vi "lab1_example_usrp_sine_signal_generator.vi"() -> ()   [LabVIEW 2014]
uses:
  <vilib>/measure/maspectr.llb/Power Spectrum and PSD Export Mode.ctl
  <vilib>/Analysis/1siggen.llb/Ramp Pattern by Samples.vi
  sub_var_stop.vi
  <instrlib>/niUSRP/niUSRP Fetch Rx Data (CDB Cluster).vi
  <vilib>/measure/maspectr.llb/FFT Power Spectrum and PSD for 1 Chan (CDB).vi
  <instrlib>/niUSRP/niUSRP Write Tx Data (CDB Cluster).vi
  <vilib>/Analysis/NI_AALBase.lvlib
  <vilib>/measure/NI_MAPro.lvlib
panel:
  out "coerced gain":dbl format="%#_6f"
  in  "number of samples":i64=20000
  out "coerced carrier frequency":dbl=915000000.0 format="%#_6p"
  out "coerced IQ rate":dbl=200000.0 format="%#_6p"
  in  "gain 2":dbl format="%#_6f"
  in  "gain":dbl format="%#_6f"
  in  "carrier frequency":dbl=915000000.0 format="%#_6p"
  in  "IQ rate":dbl=200000.0 format="%#_6p"
  in  "device names 2":refnum<k15>="192.168.10.2"
  in  "device names":refnum<k15>="192.168.10.2"
  out "Power Spectrum graph":cluster{"f0":dbl, "df":dbl, "magnitude":dbl[]}(graph)={"f0"=-0.5, "df"=5e-05, "magnitude"=[]}
  out "Sine wave":dbl[](graph)
  in  "duration":dbl=0.02 format="%#_13g"
  in  "frequency":dbl=10000.0 format="%#_13g"
  in  "stop":bool
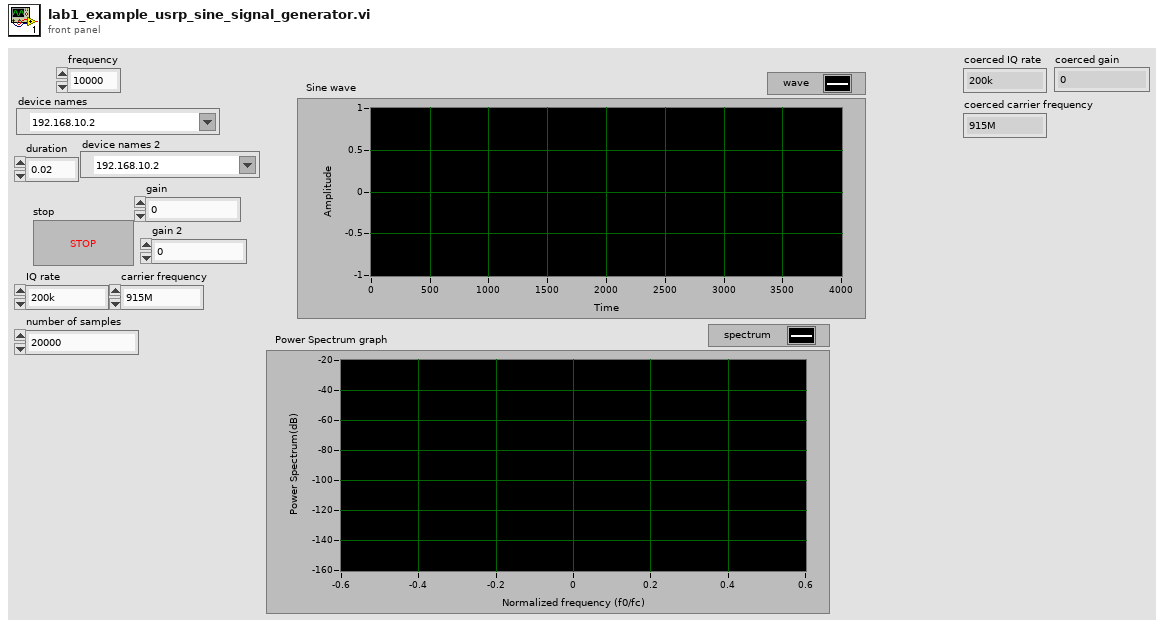
[diagram p1: front panel]
types:
  T1 = typedef "NI_MAPro.lvlib/Power Spectrum and PSD Export Mode.ctl" = u16
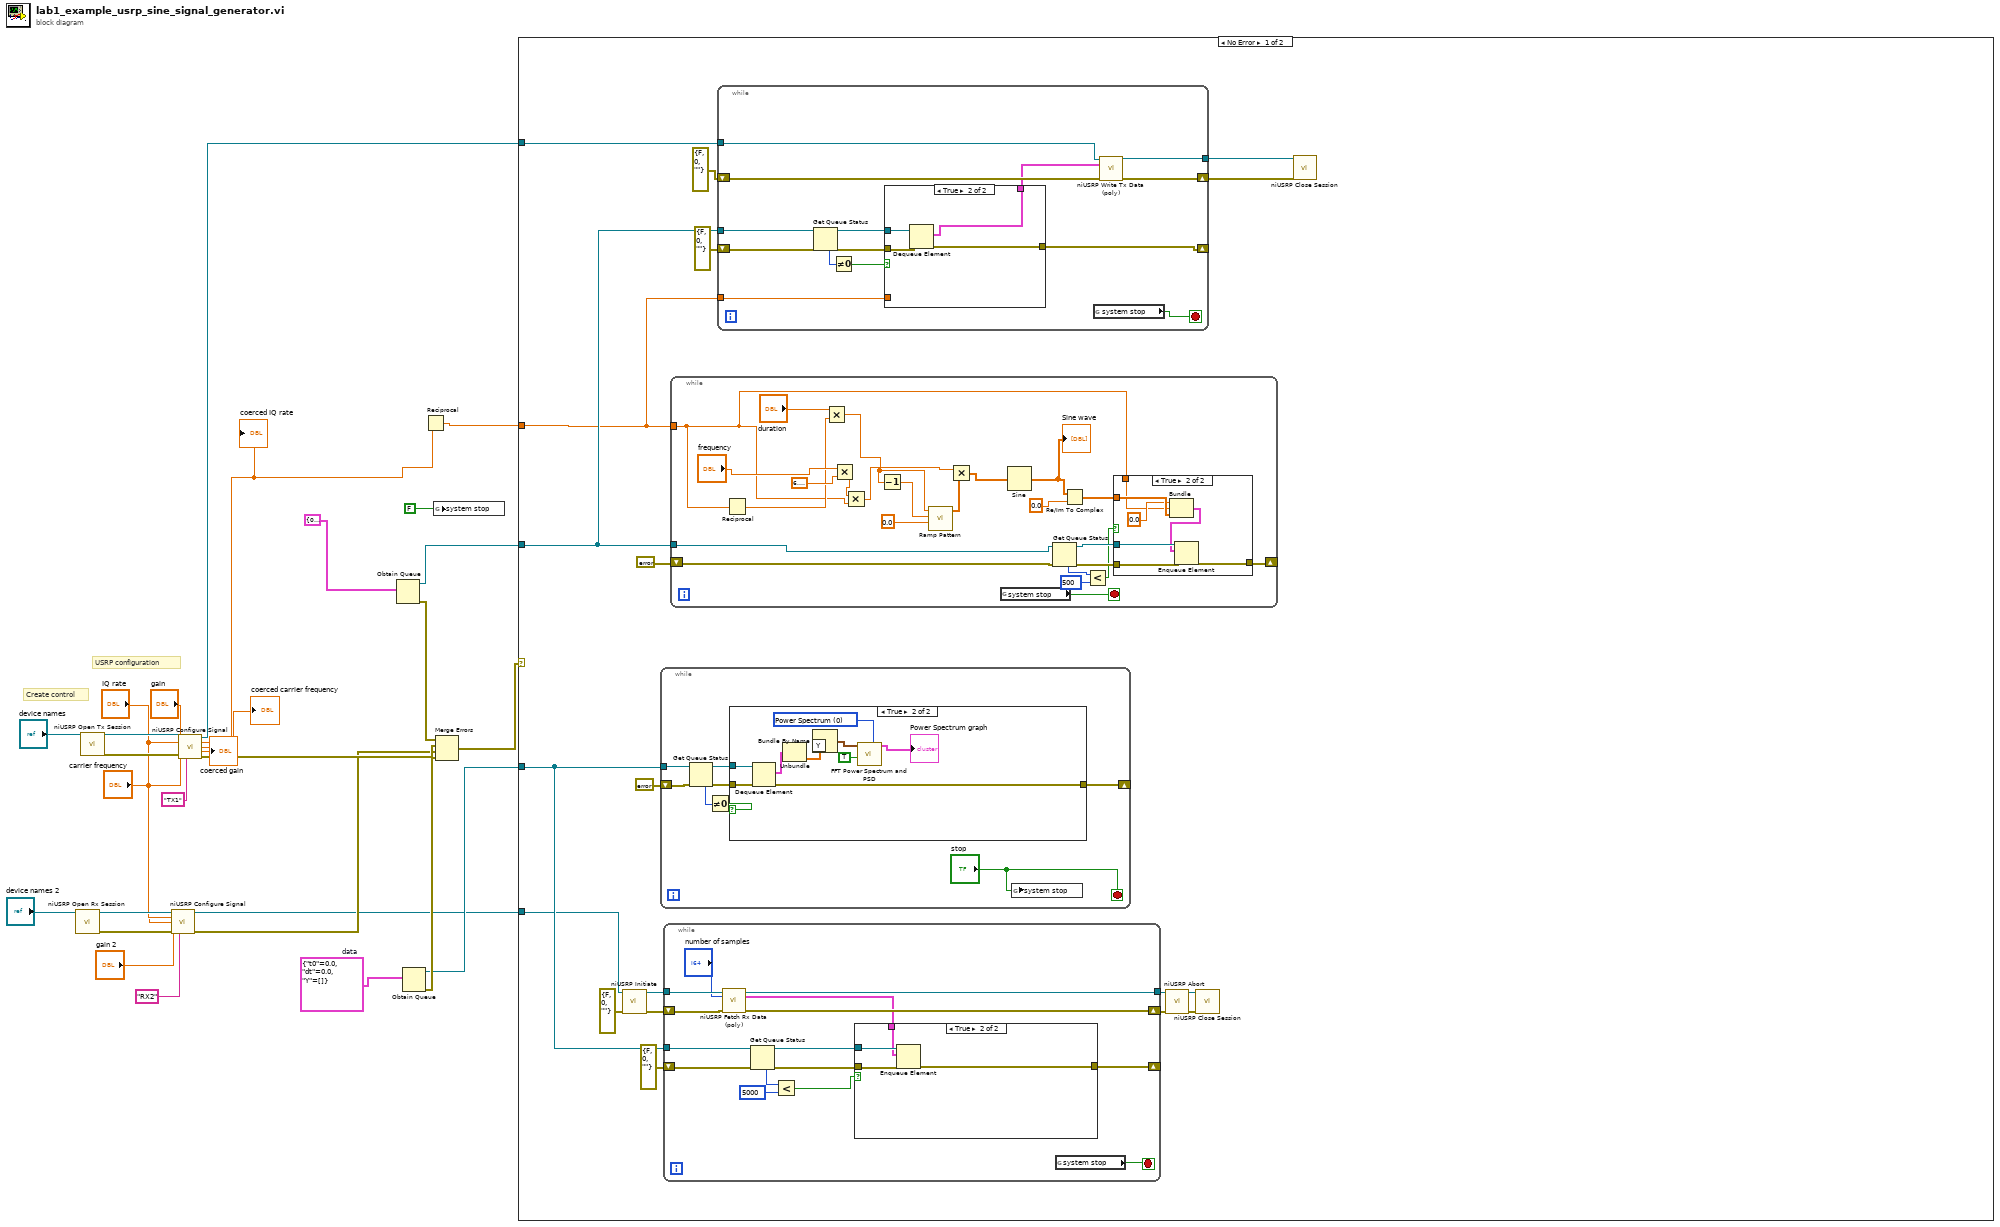
[diagram p0: block diagram]
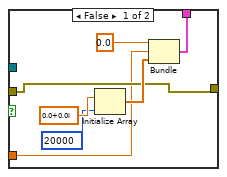
[diagram p3: hidden frame]
diagram:
  w9 = cluster{"t0":dbl, "dt":dbl, "Y":cdb[]} {"t0"=0.0, "dt"=0.0, "Y"=[]}  # data
  # "Create control"
  # "USRP configuration"
  n1 = call <instrlib>:"niUSRP Open Rx Session.vi"("device names"="device names 2") -> ("session handle out"=w24:refnum<k15>, "error out"=w23:errorcluster)  [unwired: 13 in]
  n2 = call <instrlib>:"niUSRP Open Tx Session.vi"("device names"="device names") -> ("session handle out"=w26:refnum<k15>, "error out"=w25:errorcluster)  [unwired: 13 in]
  n3 = call <instrlib>:"niUSRP Configure Signal.vi"("session handle"=w24, "IQ rate"="IQ rate", "carrier frequency"="carrier frequency", "gain"="gain 2", "error in (no error)"=w23, "active antenna"="RX2") -> ("session handle out"=w6:refnum<k15>, "error out"=w12:errorcluster)  [unwired: 5 in, 3 out]
  n4 = call <instrlib>:"niUSRP Configure Signal.vi"("session handle"=w26, "IQ rate"="IQ rate", "carrier frequency"="carrier frequency", "gain"="gain", "error in (no error)"=w25, "active antenna"="TX1") -> ("session handle out"=w5:refnum<k15>, "coerced IQ rate"=w2:dbl, "coerced carrier frequency"=→"coerced carrier frequency":dbl, "coerced gain"=→"coerced gain":dbl, "error out"=w13:errorcluster)  [unwired: 5 in]
  "coerced IQ rate" <- w2
  n5 = Obtain Queue(element data type=cluster{"t0":dbl, "dt":dbl, "Y":cdb[]} {"t0"=0.0, "dt"=1.0, "Y"=[]} ("data")) -> (queue out=w27:refnum<queue>, error out=w14:errorcluster)  [unwired: 4 in, 1 out]
  n6 = Obtain Queue(element data type=w9) -> (queue out=w7:refnum<queue>, error out=w8:errorcluster)  [unwired: 4 in, 1 out]
  n7 = Reciprocal(x=w2) -> (1/x=w4:dbl)
  n8 = global write "sub_var_stop.vi" "system stop"(FALSE) -> ()
  n9 = Merge Errors(w14, w13, w12, w8) -> (w10:errorcluster)
  n10 = case shown="No Error" w10 {
    tunnel: w27 -> [w31 _]
    tunnel: w7 -> [w35 _]
    tunnel: w6 -> [w33 _]
    tunnel: w5 -> [w32 _]
    tunnel: w4 -> [w29 _]
    frame No Error {
      n11 = call <instrlib>:"niUSRP Initiate.vi"("session handle"=w33, "error in (no error)"=errorcluster {"status"=FALSE, "code"=0, "source"=""}) -> ("session handle out"=w43:refnum<k15>, "error out"=w42:errorcluster)  [unwired: 12 in]
      n12 = while {
        tunnel: w35 -> [w99]
        shift-right: [w93] -> _
        shift-left: errorcluster {"status"=FALSE, "code"=0, "source"=""} ("error out") -> [w98]
        stop <- "stop" stop-if-true
        n13 = Get Queue Status(queue=w99, error in (no error)=w98) -> (queue out=w95:refnum<queue>, error out=w94:errorcluster, # elements in queue=w97:i32)  [unwired: 1 in, 5 out]
        n14 = Not Equal To 0?(x=w97) -> (x != 0?=w96:bool)
        n15 = case shown="True" w96 {
          tunnel: w95 -> [_ w110]
          tunnel: w94 -> [w101 w109]
          tunnel: [w101 w108] -> w93
          frame False {
          }
          frame True {
            w104 = T1 0 items=["Power Spectrum", "Power Spectral Density"] ("export mode")
            n16 = Dequeue Element(queue=w110, error in (no error)=w109) -> (element=w103:cluster{"t0":dbl, "dt":dbl, "Y":cdb[]}, error out=w108:errorcluster)  [unwired: 1 in, 2 out]
            n17 = Unbundle "Unbundle"(w103) -> ("Y"=w102:cdb[])  [unwired: 2 out]
            n18 = Bundle By Name("Y"=w102) -> (w107:waveform(cdb))  [unwired: 1 in]
            n19 = call-poly <vilib>:"FFT Power Spectrum and PSD.vi"("export mode"=w104, "dB On (F)"=TRUE, "time signal"=w107) -> ("Power Spectrum / PSD"=→"Power Spectrum graph":cluster{"f0":dbl, "df":dbl, "magnitude":dbl[]})  [unwired: 5 in, 3 out]
          }
        }
        n20 = global write "sub_var_stop.vi" "system stop"("stop") -> ()
      }
      n21 = while {
        tunnel: w43 -> [w61]
        shift-right: [w57] -> w39
        shift-left: w42 -> [w60]
        tunnel: [w58] -> w38
        tunnel: w35 -> [w56]
        shift-right: [w48] -> _
        shift-left: errorcluster {"status"=FALSE, "code"=0, "source"=""} ("error out") -> [w55]
        stop <- w62 stop-if-true
        n22 = call-poly <instrlib>:"niUSRP Fetch Rx Data (poly).vi"("session handle"=w61, "number of samples"="number of samples", "error in (no error)"=w60) -> ("session handle out"=w58:refnum<k15>, "data"=w49:cluster{"t0":dbl, "dt":dbl, "Y":cdb[]}, "error out"=w57:errorcluster)  [unwired: 9 in, 1 out]
        n23 = Get Queue Status(queue=w56, error in (no error)=w55) -> (queue out=w51:refnum<queue>, error out=w50:errorcluster, # elements in queue=w54:i32)  [unwired: 1 in, 5 out]
        n24 = Less?(x=w54, y=5000) -> (x < y?=w52:bool)
        n25 = case shown="True" w52 {
          tunnel: w51 -> [_ w67]
          tunnel: w50 -> [w63 w66]
          tunnel: w49 -> [_ w65]
          tunnel: [w63 w64] -> w48
          frame False {
          }
          frame True {
            n26 = Enqueue Element(queue=w67, element=w65, error in (no error)=w66) -> (error out=w64:errorcluster)  [unwired: 1 in, 2 out]
          }
        }
        n27 = global read "sub_var_stop.vi" "system stop"() -> (w62:bool)
      }
      n28 = while {
        tunnel: w31 -> [w130]
        shift-right: [w128] -> _
        shift-left: errorcluster {"status"=FALSE, "code"=0, "source"=""} ("error out") -> [w126]
        tunnel: w29 -> [w111]
        stop <- w134 stop-if-true
        n29 = Reciprocal(x=w111) -> (1/x=w112:dbl)
        n30 = Multiply(x="duration", y=w112) -> (x*y=w117:dbl)
        n31 = Multiply(x="frequency", y=6.283185307179586) -> (x*y=w120:dbl)
        n32 = Multiply(x=w120, y=w111) -> (x*y=w119:dbl)
        n33 = Decrement(x=w117) -> (x-1=w132:dbl)
        n34 = call-poly <vilib>:"Ramp Pattern.vi"("start"=0.0, "end"=w132, "samples"=w117) -> ("Ramp Pattern"=w131:dbl[])  [unwired: 7 in, 1 out]
        n35 = Multiply(x=w119, y=w131) -> (x*y=w116:dbl[])
        n36 = global read "sub_var_stop.vi" "system stop"() -> (w134:bool)
        n37 = Sine(x=w116) -> (sin(x)=w113:dbl[])
        "Sine wave" <- w113
        n38 = Get Queue Status(queue=w130, error in (no error)=w126) -> (queue out=w129:refnum<queue>, error out=w127:errorcluster, # elements in queue=w125:i32)  [unwired: 1 in, 5 out]
        n39 = Re/Im To Complex(1:0.0 ("start"), 2:w113) -> (0:w114:cdb[])
        n40 = Less?(x=w125, y=500) -> (x < y?=w123:bool)
        n41 = case shown="True" w123 {
          tunnel: w129 -> [_ w142]
          tunnel: [w135 w141] -> w128
          tunnel: w127 -> [w135 w140]
          tunnel: w114 -> [_ w139]
          tunnel: w111 -> [_ w137]
          frame False {
          }
          frame True {
            n42 = Bundle("start"=0.0, w137, w139) -> (w136:cluster{"start":dbl, dbl, cdb[]})  [unwired: 1 in]
            n43 = Enqueue Element(queue=w142, element=w136, error in (no error)=w140) -> (error out=w141:errorcluster)  [unwired: 1 in, 2 out]
          }
        }
      }
      n44 = while {
        shift-right: [w80] -> w41
        shift-left: errorcluster {"status"=FALSE, "code"=0, "source"=""} ("error out") -> [w78]
        tunnel: [w79] -> w40
        tunnel: w32 -> [w77]
        tunnel: w31 -> [w76]
        shift-right: [w71] -> _
        shift-left: errorcluster {"status"=FALSE, "code"=0, "source"=""} ("error out") -> [w75]
        tunnel: w29 -> [w68]
        stop <- w81 stop-if-true
        n45 = Get Queue Status(queue=w76, error in (no error)=w75) -> (queue out=w70:refnum<queue>, error out=w72:errorcluster, # elements in queue=w74:i32)  [unwired: 1 in, 5 out]
        n46 = Not Equal To 0?(x=w74) -> (x != 0?=w73:bool)
        n47 = case shown="True" w73 {
          tunnel: w72 -> [w83 w92]
          tunnel: [w83 w91] -> w71
          tunnel: w70 -> [_ w90]
          tunnel: [w88 w89] -> w69
          tunnel: w68 -> [w82 _]
          frame False {
            n48 = Initialize Array(cdb 0.0+0.0i, 20000 ("dimension size")) -> (w85:cdb[])
            n49 = Bundle(0.0, w82, w85) -> (w88:cluster{dbl, dbl, cdb[]})  [unwired: 1 in]
          }
          frame True {
            n50 = Dequeue Element(queue=w90, error in (no error)=w92) -> (element=w89:cluster{"t0":dbl, "dt":dbl, "Y":cdb[]}, error out=w91:errorcluster)  [unwired: 1 in, 2 out]
          }
        }
        n51 = global read "sub_var_stop.vi" "system stop"() -> (w81:bool)
        n52 = call-poly <instrlib>:"niUSRP Write Tx Data (poly).vi"("session handle"=w77, "data"=w69, "error in (no error)"=w78) -> ("session handle out"=w79:refnum<k15>, "error out"=w80:errorcluster)  [unwired: 11 in]
      }
      n53 = call <instrlib>:"niUSRP Abort.vi"("session handle"=w38, "error in (no error)"=w39) -> ("session handle out"=w45:refnum<k15>, "error out"=w44:errorcluster)  [unwired: 12 in]
      n54 = call <instrlib>:"niUSRP Close Session.vi"("session handle"=w45, "error in (no error)"=w44) -> ()  [unwired: 13 in, 1 out]
      n55 = call <instrlib>:"niUSRP Close Session.vi"("session handle"=w40, "error in (no error)"=w41) -> ()  [unwired: 13 in, 1 out]
    }
    frame Error {
    }
  }
